vi "Pt Dist.vi"(10 "point b":cluster{"x":dbl, "y":dbl}, 11 "point a":cluster{"x":dbl, "y":dbl}) -> (3 "dist":dbl)   [LabVIEW 2019]
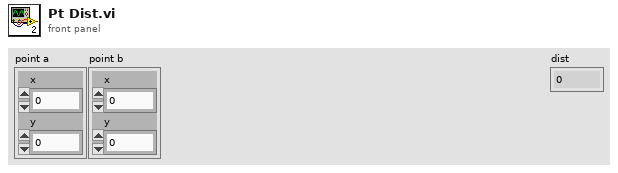
[diagram p1: front panel]
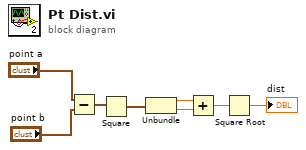
[diagram p0: block diagram]
diagram:
  n1 = Subtract(x="point a", y="point b") -> (x-y=w6:cluster{"x":dbl, "y":dbl})
  n2 = Square(x=w6) -> (x^2=w5:cluster{"x":dbl, "y":dbl})
  n3 = Unbundle(w5) -> ("x"=w4:dbl, "y"=w3:dbl)
  n4 = Add(x=w4, y=w3) -> (x+y=w2:dbl)
  n5 = Square Root(x=w2) -> (sqrt(x)=→"dist":dbl)
